vi "Draw Arrow.vi"(9 "Start Y":dbl, 10 "Start X":dbl, 11 "Vector":cluster{"r":dbl, "Theta":dbl}) -> (0 "Y":dbl[](array[numeric]), 1 "X":dbl[](array[numeric]), 3 "Points":cluster{dbl[], dbl[]})   [LabVIEW 2025]
panel:
  out "XY Graph":cluster{dbl[], dbl[]}(graph)
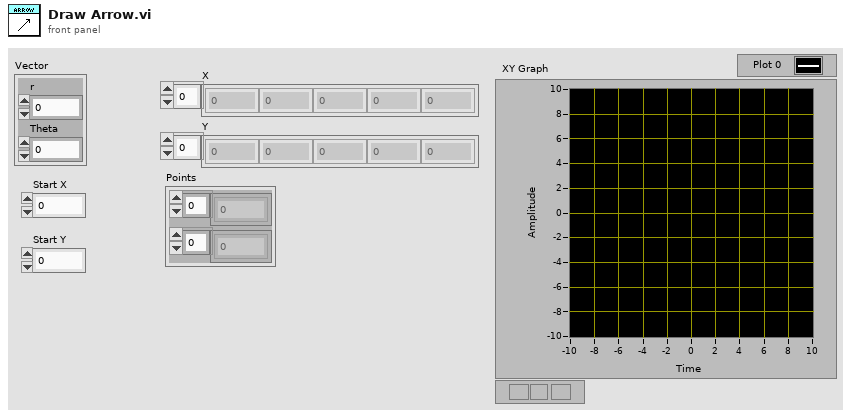
[diagram p1: front panel]
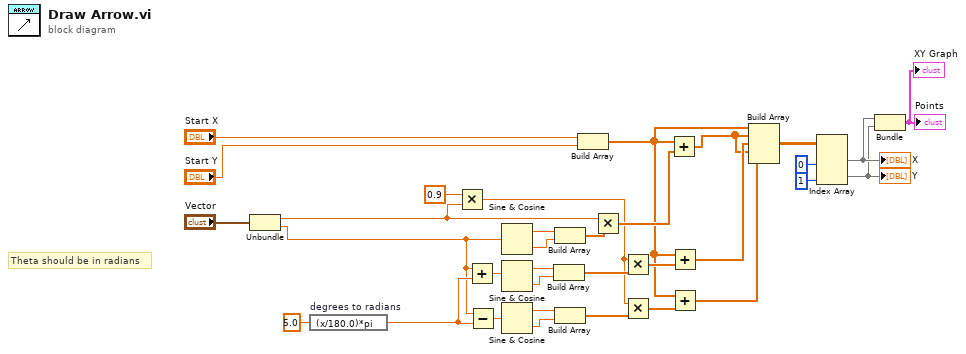
[diagram p0: block diagram]
diagram:
  # "Theta should be in radians"
  n1 = Unbundle("Vector") -> ("r"=w3:dbl, "Theta"=w1:dbl)
  n2 = expression code="(x/180.0)*pi" "degrees to radians"(5.0) -> (w4:dbl)
  n3 = Multiply(x=0.9, y=w3) -> (x*y=w6:dbl)
  n4 = Add(x=w1, y=w4) -> (x+y=w28:dbl)
  n5 = Subtract(x=w1, y=w4) -> (x-y=w27:dbl)
  n6 = Sine & Cosine(0:w1) -> (1:w26:dbl, 2:w25:dbl)
  n7 = Sine & Cosine(0:w28) -> (1:w24:dbl, 2:w22:dbl)
  n8 = Sine & Cosine(0:w27) -> (1:w23:dbl, 2:w21:dbl)
  n9 = Build Array(w24, w22) -> (w20:dbl[])
  n10 = Build Array(w26, w25) -> (w32:dbl[])
  n11 = Build Array(w23, w21) -> (w19:dbl[])
  n12 = Build Array("Start X", "Start Y") -> (w16:dbl[])
  n13 = Multiply(x=w3, y=w32) -> (x*y=w29:dbl[])
  n14 = Multiply(x=w6, y=w20) -> (x*y=w18:dbl[])
  n15 = Multiply(x=w6, y=w19) -> (x*y=w17:dbl[])
  n16 = Add(x=w16, y=w29) -> (x+y=w14:dbl[])
  n17 = Add(x=w16, y=w18) -> (x+y=w15:dbl[])
  n18 = Add(x=w16, y=w17) -> (x+y=w13:dbl[])
  n19 = Build Array(w16, w14, w15, w14, w13) -> (w12:dbl[][])
  n20 = Index Array(array=w12, index (col) #1=0 ("disabled index (col)"), index (col) #2=1 ("index (col)")) -> (element #1=w9:dbl[], element #2=w8:dbl[])  [unwired: 2 in]
  "X" <- w9
  "Y" <- w8
  n21 = Bundle(w9, w8) -> (→"Points" →"XY Graph":cluster{dbl[], dbl[]})  [unwired: 1 in]
